vi "Test Autoco.vi"() -> ()   [LabVIEW 2024]
uses:
  <vilib>/Utility/miscctls.llb/LVRangeTypeDef.ctl
  <vilib>/Utility/miscctls.llb/LVOffsetAndMultiplierTypeDef.ctl
  <vilib>/Analysis/6fits.llb/Curve Fitting Criteria.ctl
  <vilib>/Analysis/2dsp.llb/Integral Method.ctl
  <vilib>/Analysis/1siggen.llb/Ramp Pattern by Samples.vi
  <vilib>/Analysis/8numeric.llb/1D Numeric Integration.vi
  <vilib>/Analysis/1siggen.llb/Ramp Pattern by Delta.vi
  <vilib>/Analysis/NI_AALBase.lvlib
  <vilib>/Analysis/NI_AALPro.lvlib
panel:
  out "x/y 2":dbl[unit]
  out "x/y":dbl
  out "Ramp Pattern 3":dbl[](array[numeric]) caption="Motif de rampe"
  out "Graphe XY":cluster{dbl[], "Best Gaussian Fit":dbl[]}[](graph)
  out "tableau":dbl[][](array[numeric])
  out "Autoccorrélation":dbl[][](graph)
  out "Ramp Pattern 2":dbl[](array[numeric]) caption="Motif de rampe"
  out "Échelle des X.Gamme":T1
  out "result":dbl caption="résultat" format="%0.4f"
  out "Pos Curseur Y2":dbl
  out "Pos Curseur Y1":dbl
  in  "Booléen":bool=TRUE
  out "Graphe":dbl[](graph)
  out "taille(s)":i32
  out "Ramp Pattern":dbl[](array[numeric]) caption="Motif de rampe"
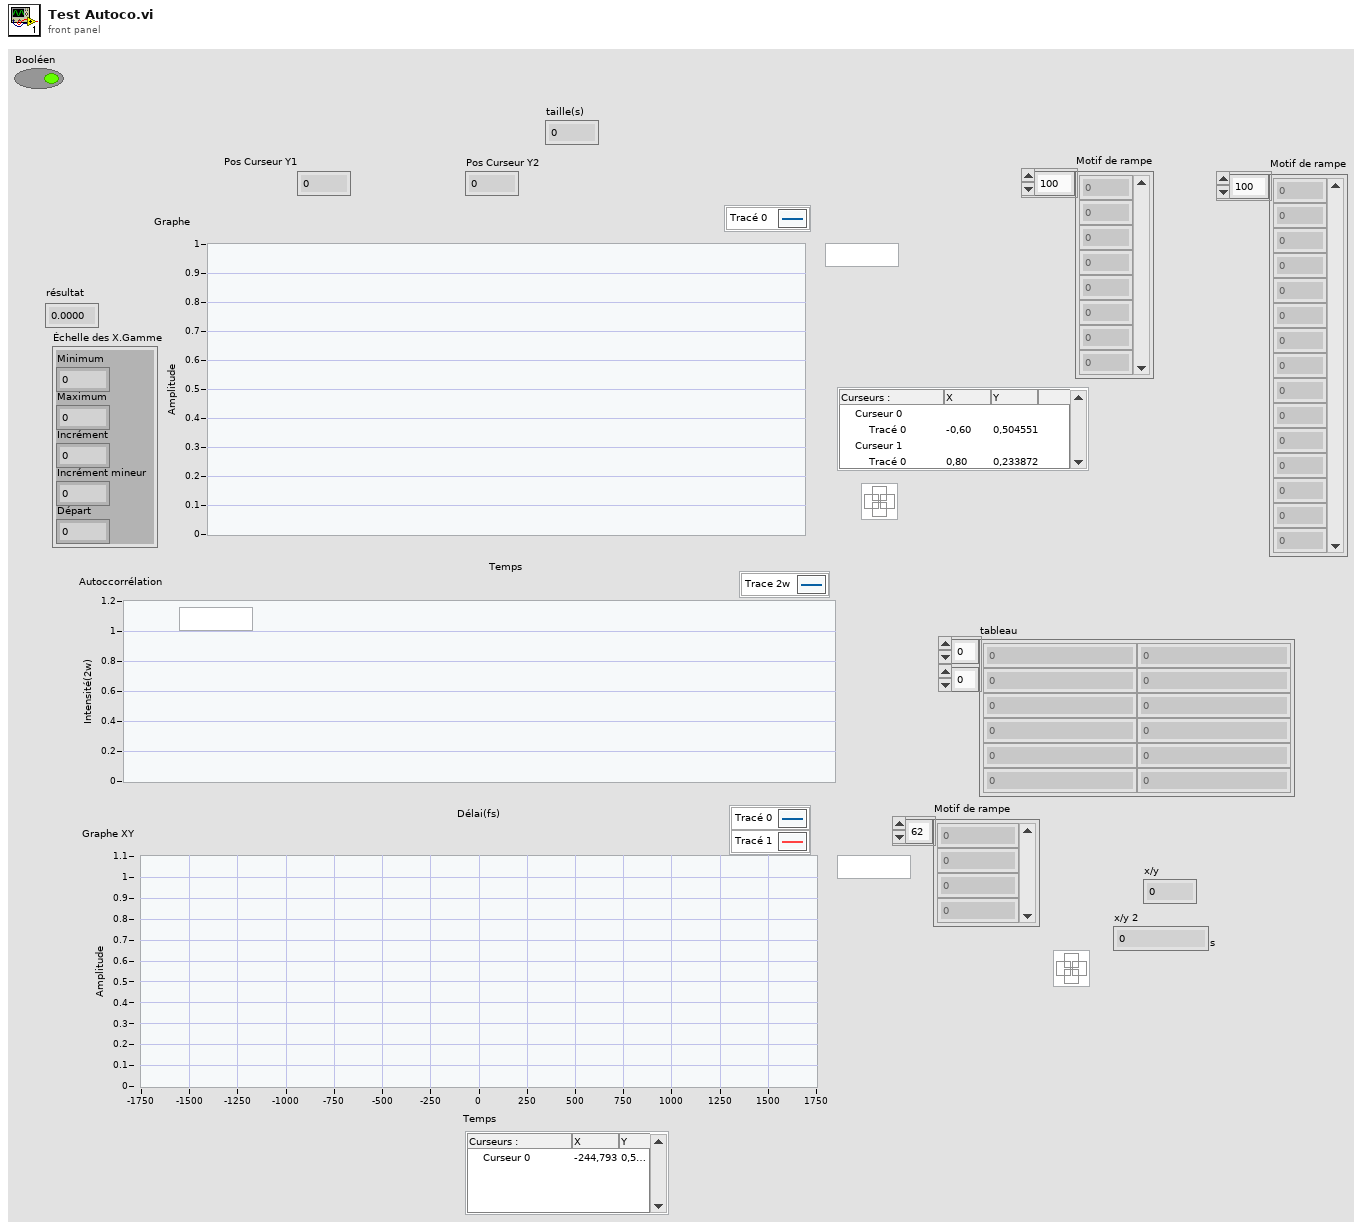
[diagram p1: front panel]
types:
  T1 = typedef "LVRangeTypeDef.ctl" = cluster{"Minimum":dbl, "Maximum":dbl, "Increment":dbl, "Minor Increment":dbl, "Start":dbl}
  T2 = typedef "NI_AALPro.lvlib/Curve Fitting Criteria.ctl" = u16
  T3 = typedef "LVOffsetAndMultiplierTypeDef.ctl" = cluster{"Offset":dbl, "Multiplier":dbl}
  T4 = typedef "NI_AALPro.lvlib/Integral Method.ctl" = i32
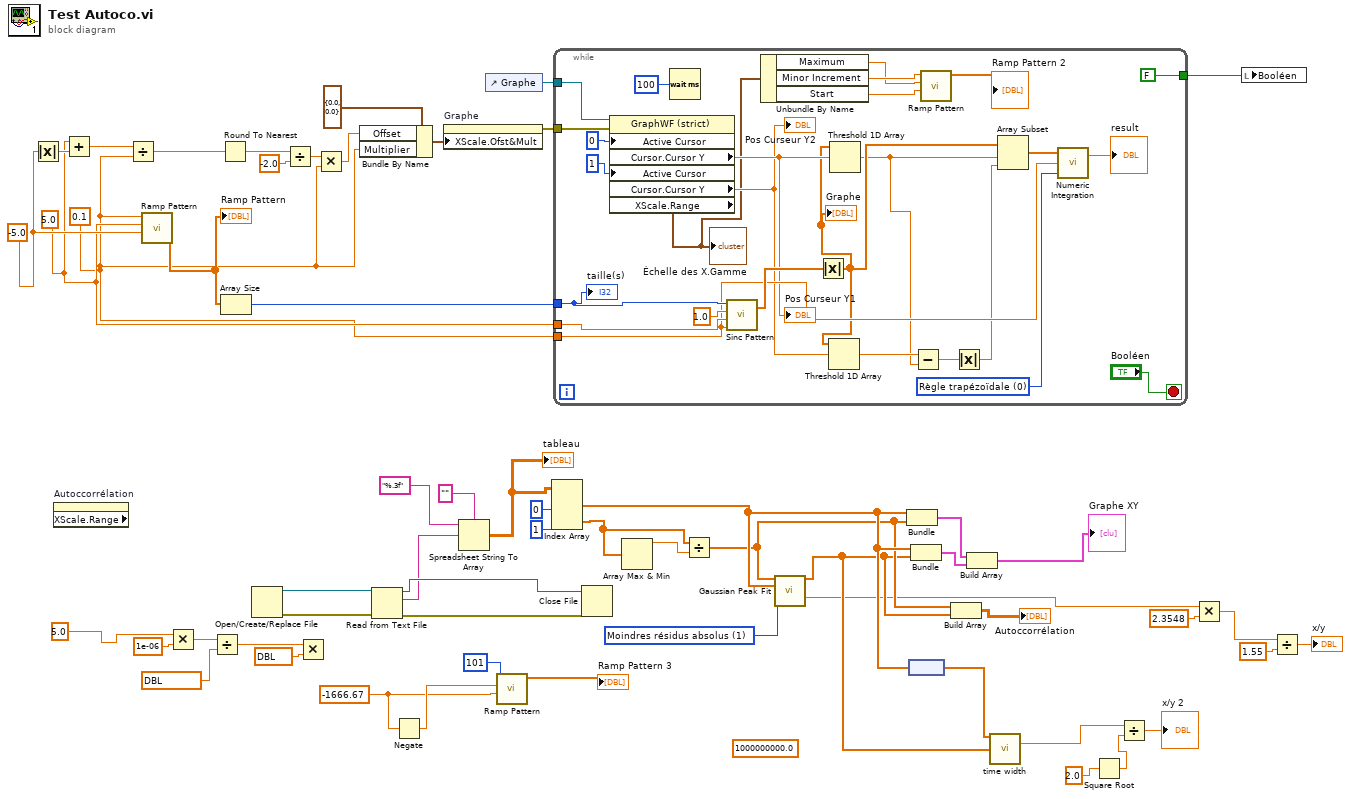
[diagram p0: block diagram]
diagram:
  (unwired) 1000000000.0
  w15 = -1666.67
  w30 = T2 1 items=["Moindres carrés", "Moindres résidus absolus", "Bicarrée"] ("method")
  w45 = 0.1 ("delta")
  w53 = -5.0 ("start")
  w51 = 5.0 ("end")
  n1 = Absolute Value(x=w53) -> (abs(x)=w52:dbl)
  n2 = property on="Autoccorrélation" class="GraphWF (strict)" props=["XScale", "Range"]() -> ()  [unwired: 2 in, 3 out]
  n3 = Add(x=w51, y=w52) -> (x+y=w50:dbl)
  n4 = Divide(x=w50, y=w45) -> (x/y=w47:dbl)
  n5 = call-poly <vilib>:"Ramp Pattern.vi"("start"=w53, "end"=w51, "delta"=w45) -> ("Ramp Pattern"=w54:dbl[])  [unwired: 6 in, 2 out]
  "Ramp Pattern" <- w54
  n6 = Multiply(x=5.0, y=1e-06) -> (x*y=w23:dbl)
  n7 = Divide(x=w23, y=ext[unit] 300000000.0) -> (x/y=w19:ext[unit])
  n8 = Round To Nearest(number=w47) -> (nearest integer value=w46:dbl)
  n9 = Array Size(array=w54) -> (size(s)=w57:i32)
  n10 = Open/Create/Replace File() -> (refnum out=w40:refnum<file>, error out=w37:errorcluster)  [unwired: 6 in, 1 out]
  n11 = Divide(x=w46, y=-2.0) -> (x/y=w48:dbl)
  n12 = Multiply(x=w19, y=ext[unit] 1000000000000000.0) -> ()  [unwired: 1 out]
  n13 = Multiply(x=w48, y=w45) -> (x*y=w44:dbl)
  n14 = Bundle By Name(cluster=T3 {"Offset"=0.0, "Multiplier"=0.0} ("Échelle des X.Offset et multiplicateur"), "Offset"=w44, "Multiplier"=w45) -> (w55:T3)
  n15 = Read from Text File(file (use dialog)=w40, error in=w37) -> (refnum out=w39:refnum<file>, text=w36:string, error out=w38:errorcluster)  [unwired: 2 in, 1 out]
  n16 = Negate(x=w15) -> (-x=w17:dbl)
  n17 = property on="Graphe" class="GraphWF (strict)"("XScale.Ofst&Mult"=w55) -> (error out=w43:errorcluster)  [unwired: 2 in, 1 out]
  n18 = Spreadsheet String To Array(delimiter (Tab)="" ("séparateur (Tabulation)"), format string="%.3f" ("chaîne de format"), spreadsheet string=w36) -> (array=w33:dbl[][])  [unwired: 1 in]
  "tableau" <- w33
  n19 = control-ref of="Graphe"() -> (w42:refnum<vi>)
  n20 = call-poly <vilib>:"Ramp Pattern.vi"("start"=w15, "end"=w17, "samples"=101) -> ("Ramp Pattern"=→"Ramp Pattern 3":dbl[])  [unwired: 7 in, 1 out]
  n21 = Index Array(array=w33, index (col) #1=0 ("indice désactivé (col)"), index (col) #2=1 ("indice (col)")) -> (element #1=w14:dbl[], element #2=w25:dbl[])  [unwired: 2 in]
  n22 = while {
    tunnel: w57 -> [w83]
    tunnel: w51 -> [w82]
    tunnel: w45 -> [w73]
    tunnel: w43 -> [w78]
    tunnel: w42 -> [w75]
    tunnel: [FALSE] -> w41
    stop <- "Booléen" stop-if-true
    w72 = T4 0 items=["Règle trapézoïdale", "Règle de Simpson", "Règle de Simpson 3/8", "Règle de Bode"] ("integration method")
    n23 = property on="Nœud de propriété" class="GraphWF (strict)"(reference=w75, error in=w78, "Active Cursor"=u32 0 ("Curseur actif"), "Active Cursor"=u32 1 ("Curseur actif")) -> ("Cursor.Cursor Y"=w70:dbl, "Cursor.Cursor Y"=w69:dbl, "XScale.Range"=w62:T1)  [unwired: 2 out]
    "Pos Curseur Y1" <- w70
    "Pos Curseur Y2" <- w69
    "Échelle des X.Gamme" <- w62
    n24 = Wait (ms)(milliseconds to wait=u32 100 ("attente (ms)")) -> ()  [unwired: 1 out]
    n25 = call <vilib>:"Sinc Pattern.vi"("delta t"=w73, "delay"=w82, "amplitude"=1.0, "samples"=w83) -> ("Sinc Pattern"=w81:dbl[])  [unwired: 1 out]
    n26 = Unbundle By Name(w62) -> ("Maximum"=w59:dbl, "Minor Increment"=w60:dbl, "Start"=w61:dbl)
    n27 = Absolute Value(x=w81) -> (abs(x)=w68:dbl[])
    "Graphe" <- w68
    n28 = Threshold 1D Array(2:w69, 3:w68) -> (0:w66:dbl)  [unwired: 1 in]
    n29 = Threshold 1D Array(2:w70, 3:w68) -> (0:w65:dbl)  [unwired: 1 in]
    n30 = Subtract(x=w66, y=w65) -> (x-y=w64:dbl)
    n31 = call-poly <vilib>:"Ramp Pattern.vi"("start"=w61, "end"=w59, "delta"=w60) -> ("Ramp Pattern"=→"Ramp Pattern 2":dbl[])  [unwired: 6 in, 2 out]
    n32 = Absolute Value(x=w64) -> (abs(x)=w63:dbl)
    n33 = Array Subset(array=w68, index=w65, length=w63) -> (w67:dbl[])
    n34 = call-poly <vilib>:"Numeric Integration.vi"("integration method"=w72, "dt"=w73, "Input Array"=w67) -> ("result"=→"result":dbl)  [unwired: 1 out]
    "taille(s)" <- w83
  }
  n35 = Close File(refnum=w39, error in=w38) -> ()  [unwired: 2 out]
  n36 = Array Max & Min(array=w25) -> (max value=w26:dbl)  [unwired: 3 out]
  n37 = Divide(x=w25, y=w26) -> (x/y=w9:dbl[])
  n38 = call <vilib>:"Gaussian Peak Fit.vi"("Y"=w9, "X"=w14, "method"=w30) -> ("Best Gaussian Fit"=w8:dbl[], "standard deviation"=w3:dbl)  [unwired: 6 in, 5 out]
  n39 = Bundle(w14, w9) -> (w29:cluster{dbl[], dbl[]})  [unwired: 1 in]
  n40 = node(w14) -> (w13:dbl[unit][])
  n41 = Bundle(w14, "Best Gaussian Fit"=w8) -> (w28:cluster{dbl[], "Best Gaussian Fit":dbl[]})  [unwired: 1 in]
  n42 = Build Array(w9, w8) -> (→"Autoccorrélation":dbl[][])
  n43 = Build Array(w29, w28) -> (→"Graphe XY":cluster{dbl[], "Best Gaussian Fit":dbl[]}[])
  n44 = call <userlib>:"time width.vi"("time"=w13, "y vector"=w8) -> ("FWHM t"=w12:dbl[unit])  [unwired: 12 in, 1 out]
  n45 = Square Root(x=2.0) -> (sqrt(x)=w10:dbl)
  n46 = Divide(x=w12, y=w10) -> (x/y=→"x/y 2":dbl[unit])
  n47 = Multiply(x=w3, y=2.3548) -> (x*y=w5:dbl)
  n48 = local write "Booléen"(w41) -> ()
  n49 = Divide(x=w5, y=1.55) -> (x/y=→"x/y":dbl)
